vi "Turn From Angle.vi"(11 "Desired Angle":dbl) -> (3 "Done?":bool)   [LabVIEW 2016]
doc: "Turns the robot a given amount of degrees from where the robot is currently at."
uses:
  \\LAKOTAROBOTICS\Public/Share2_BigFiles/Machine Committee/Controls/_Controls 2017/2017 Robot Project/Robot Values.vi
  <vilib>/addons/control/pid/pid.llb/PID (DBL).vi
  <vilib>/addons/control/pid/NI_PID_pid.lvlib
panel:
  in  "reinitialize? (F)":bool
  in  "PID gains":T1={"proportional gain (Kc)"=1.0, "integral time (Ti, min)"=0.01, "derivative time (Td, min)"=0.0} {"derivative time (Td, min)" format="%.3f"; "integral time (Ti, min)" format="%.3f"; "proportional gain (Kc)" format="%.3f"}
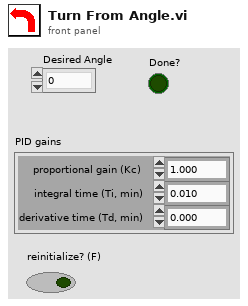
[diagram p1: front panel]
types:
  T1 = cluster{"proportional gain (Kc)":dbl, "integral time (Ti, min)":dbl, "derivative time (Td, min)":dbl}
  T2 = typedef "Robot Values.ctl" = cluster{"Robot Drive":cluster{"Left Motor Power":dbl, "Right Motor Power":dbl, "Left Encoder Value":dbl, "Right Encoder Value":dbl}, "Sensors":cluster{"Gyro Angle":dbl}}
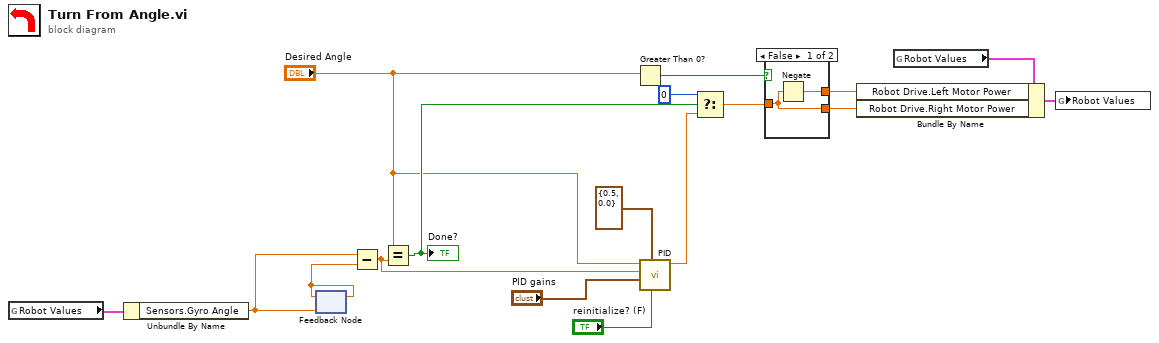
[diagram p0: block diagram]
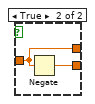
[diagram p2: hidden frame]
diagram:
  n1 = global read "Robot Values.vi" "Robot Values"() -> (w13:T2)
  n2 = Unbundle By Name(w13) -> ("Sensors.Gyro Angle"=w14:dbl)
  n3 = feedback #1(w14) -> (w15:dbl)
  n4 = feedback-in #1(w15) -> ()
  n5 = Subtract(x=w14, y=w15) -> (x-y=w2:dbl)
  n6 = Equal?(x="Desired Angle", y=w2) -> (x = y?=w16:bool)
  "Done?" <- w16
  n7 = Greater Than 0?(x="Desired Angle") -> (x > 0?=w17:bool)
  n8 = call-poly <vilib>:"PID.vi"("reinitialize? (F)"="reinitialize? (F)", "output range"=cluster{"output high":dbl, "output low":dbl} {"output high"=0.5, "output low"=0.0}, "PID gains"="PID gains", "process variable"=w2, "setpoint"="Desired Angle") -> ("output"=w1:dbl)  [unwired: 5 in, 1 out]
  n9 = Select(t=0, s=w16, f=w1) -> (s? t:f=w7:dbl)
  n10 = case shown="False" w17 {
    tunnel: [w18 w21] -> w10
    tunnel: [w19 w20] -> w9
    tunnel: w7 -> [w19 w21]
    frame False {
      n11 = Negate(x=w19) -> (-x=w18:dbl)
    }
    frame True {
      n12 = Negate(x=w21) -> (-x=w20:dbl)
    }
  }
  n13 = global read "Robot Values.vi" "Robot Values"() -> (w11:T2)
  n14 = Bundle By Name(cluster=w11, "Robot Drive.Left Motor Power"=w10, "Robot Drive.Right Motor Power"=w9) -> (w12:T2)
  n15 = global write "Robot Values.vi" "Robot Values"(w12) -> ()
